vi "Generate Status Message From Number.vi"(11 "HMI Message":u8) -> (3 "String":string)   [LabVIEW 2015]
panel:
  in  "HMI Messages":string[](array[string])=["No recipe selected - surpervisor to load recipe\t\t", "Emergency stop active - supervisor to reset alarm\t\t", "Press physical reset button and then clear E-stop alarm again\t\t", "Part failed - supervisor to reset station\t\t", "Part passed - operator to open hand clamp\t\t", "Waiting for hand clamp to be opened\t\t", "Waiting for start button to be pressed\t\t", "Waiting for two-hand start to be pressed\t\t", "Waiting for belt slide button to be fully depressed\t\t", "Tug test requires both start buttons to be pressed and held\t\t", "Remove first sonotrode and perform required welds\t\t", "Remove second sonotrode and perform required welds\t\t", "Remove third sonotrode and perform required weld\t\t", "Incorrect sonotrode removed from holster\t\t", "Not all the sonotrodes are in their holster\t\t", "More than one sonotrode removed from holster\t\t", "Stamp cylinder movement timeout - part not marked correctly\t\t", "Stamp cylinder movement timeout - cylinder not retracting correctly\t\t", "Clamp open - close clamp and press start button again\t\t", "Pivot cylinder actuate movement timeout\t\t", "Pivot cylinder retract movement timeout\t\t", "Tug test cylinder actuate movement timeout\t\t", "Tug test cylinder retract movement timeout\t\t", "Tug test cylinder not in home position, press two-hand start to home cylinder\t\t"]
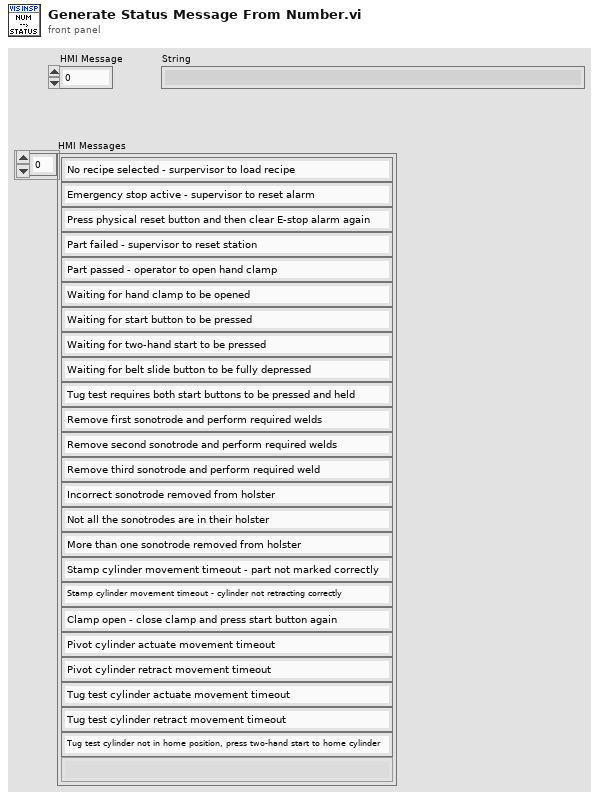
[diagram p1: front panel]
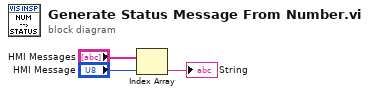
[diagram p0: block diagram]
diagram:
  n1 = Index Array(array="HMI Messages", index="HMI Message") -> (element=→"String":string)
